vi "Koheras_Seed_Laser_Power.vi"(8 "error in":errorcluster, 10 "laserPower":i32, 11 "VISA resource name in":refnum<visa-resource-name>) -> (0 "error out":errorcluster, 2 "Return":string[](array[string]), 3 "VISA resource name out":refnum<visa-resource-name>)   [LabVIEW 2011]
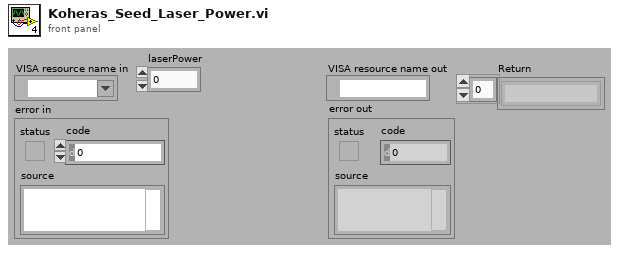
[diagram p1: front panel]
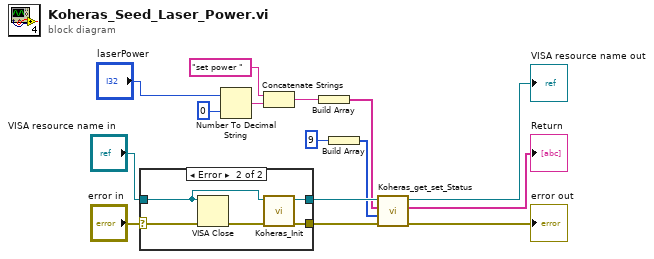
[diagram p0: block diagram]
diagram:
  n1 = case shown="Error" "error in" {
    selector: "error in" -> [w16 w21]
    tunnel: "VISA resource name in" -> [w17 w20]
    tunnel: [w16 w19] -> w6
    tunnel: [w17 w18] -> w5
    frame No Error {
    }
    frame Error {
      n2 = VISA Close(VISA resource name=w20, error in (no error)=w21) -> (error out=w22:errorcluster)
      n3 = call "Koheras_Init.vi"("error in"=w22, "VISA resource name"=w20) -> ("error out"=w19:errorcluster, "VISA resource name out"=w18:refnum<visa-resource-name>)  [unwired: 8 in]
    }
  }
  n4 = Number To Decimal String(number="laserPower", width (-)=i16 0) -> (decimal integer string=w15:string)
  n5 = Concatenate Strings("set power " ("string"), w15) -> (w13:string)
  n6 = Build Array(w13) -> (w2:string[])
  n7 = Build Array(9 ("new element/subarray")) -> (w1:i32[])
  n8 = call "Koheras_get_set_Status.vi"("error in"=w6, "Array 2"=w1, "Array"=w2, "VISA resource name in"=w5) -> ("error out"=→"error out":errorcluster, "Return"=→"Return":string[], "VISA resource name out"=→"VISA resource name out":refnum<visa-resource-name>)  [unwired: 5 in]
